vi "Zad1.vi"() -> ()   [LabVIEW 2015]
panel:
  out "String":string
  in  "stop":bool
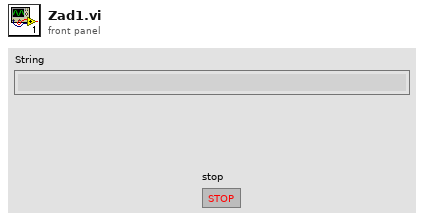
[diagram p1: front panel]
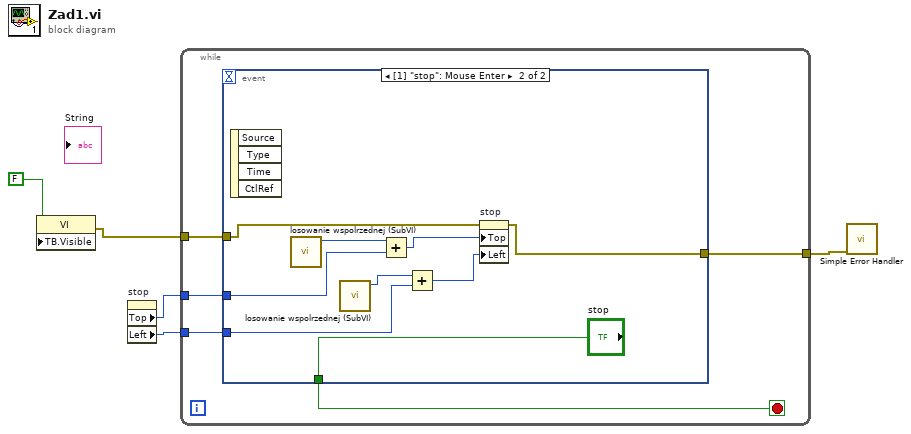
[diagram p0: block diagram]
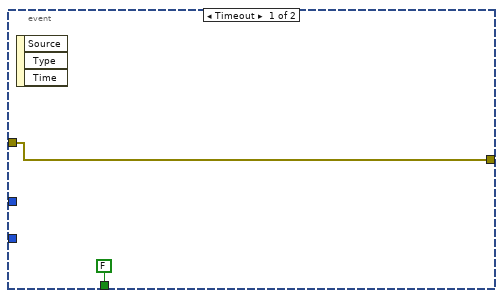
[diagram p2: hidden frame]
diagram:
  n1 = property class="VI"("TB.Visible"=FALSE ("Tool Bar:Visible")) -> (error out=w1:errorcluster)  [unwired: 2 in, 1 out]
  n2 = property on="stop" class="Bool"() -> ("Top"=w4:i32, "Left"=w3:i32)  [unwired: 2 in, 2 out]
  n3 = while {
    tunnel: w1 -> [w10]
    tunnel: [w8] -> w5
    tunnel: w4 -> [w7]
    tunnel: w3 -> [w6]
    stop <- w9 stop-if-true
    n4 = event shown="[1] \"stop\": Mouse Enter" {
      selector: _ -> [_ _]
      dyn-events: _ -> [_ _]
      timeout: _ -> [_ _]
      tunnel: w10 -> [w11 w20]
      tunnel: [FALSE ("stop") "stop"] -> w9
      tunnel: [w11 w19] -> w8
      tunnel: w7 -> [_ w13]
      tunnel: w6 -> [_ w14]
      event Timeout {
        n5 = event-data() -> ()  [unwired: 1 in, 3 out]
      }
      event "stop": Mouse Enter {
        n6 = event-data() -> ()  [unwired: 1 in, 4 out]
        n7 = call "losowanie wspolrzednej (SubVI).vi"() -> ("Numeric"=w18:i32)  [unwired: 11 in]
        n8 = call "losowanie wspolrzednej (SubVI).vi"() -> ("Numeric"=w16:i32)  [unwired: 11 in]
        n9 = Add(x=w18, y=w13) -> (x+y=w17:i32)
        n10 = Add(x=w16, y=w14) -> (x+y=w15:i32)
        n11 = property on="stop" class="Bool"(error in=w20, "Top"=w17, "Left"=w15) -> (error out=w19:errorcluster)  [unwired: 1 in, 1 out]
      }
    }
  }
  n12 = call <vilib>:"Simple Error Handler.vi"("error in (no error)"=w5) -> ()  [unwired: 4 in, 5 out]
